vi "Read Logger Config.vi"(8 "error in (no error)":errorcluster, 11 "Step Configuration in":refnum<class "Step Configuration.lvclass">) -> (0 "error out":errorcluster, 2 "Logger.lvlib:Logger Configuration.lvclass":refnum<class "Logger Configuration.lvclass">, 3 "Step Configuration out":refnum<class "Step Configuration.lvclass">)   [LabVIEW 2017, in "Measurement Actor.lvlib" / "Step Configuration.lvclass"]
uses:
  Step Configuration.lvclass
  Logger/config/Logger Configuration.lvclass
  Step Configuration.lvclass/Step Configuration.ctl
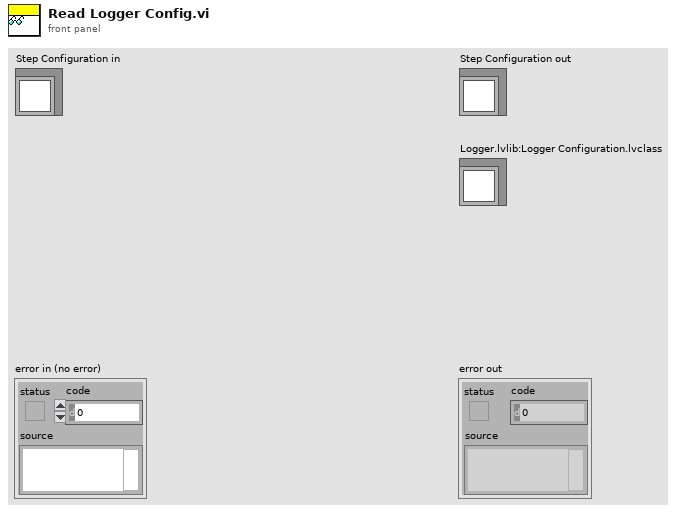
[diagram p1: front panel]
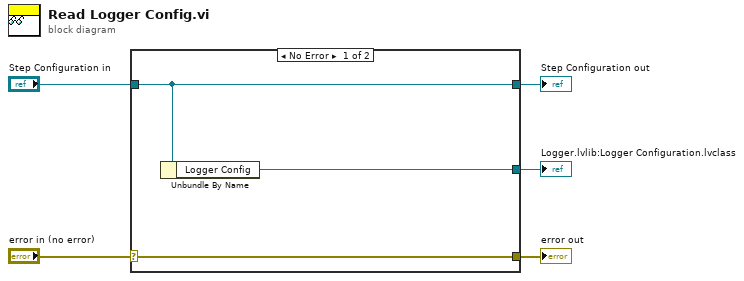
[diagram p0: block diagram]
diagram:
  n1 = case shown="No Error" "error in (no error)" {
    selector: "error in (no error)" -> [w8 w9]
    tunnel: [w8 w9] -> w4
    tunnel: [w7 w10] -> w2
    tunnel: "Step Configuration in" -> [w7 w10]
    tunnel: [w6 _] -> w1
    frame No Error {
      n2 = Unbundle By Name(w7) -> ("Logger Config"=w6:refnum<class "Logger Configuration.lvclass">)
    }
    frame Error {
    }
  }
  "error out" <- w4
  "Step Configuration out" <- w2
  "Logger.lvlib:Logger Configuration.lvclass" <- w1
